vi "Get IP.vi"(8 "error in (no error)":errorcluster, 10 "ID":string, 11 "Guardian List in":refnum<class "Guardian List.lvclass">) -> (0 "error out":errorcluster, 2 "IP":string, 3 "Guardian List out":refnum<class "Guardian List.lvclass">)   [LabVIEW 2026, in "TALOS.lvlib" / "Classes.lvlib" / "Guardian List.lvclass"]
uses:
  Guardian List.lvclass
  Guardian List.lvclass/Guardian List.ctl
  Ancestor/Ancestor/Ancestor.lvclass/Ancestor.ctl
  FGV/Error Memory/Get Error Description.vi
  Support VIs/Get PC name.vi
  Ancestor/Ancestor/Read ID.vi
  Support VIs/Get Class Name.vi
  <vilib>/Utility/error.llb/Clear Errors.vi
  FGV/Error Memory/Error Memory Core.vi
  <vilib>/AdvancedString/Delimited String to 1D String Array.vi
  <vilib>/AdvancedString/Delimited String to 1D String Array (string).vi
  Support VIs/Circus Root Path.vi
  FGV/Error Memory/Error Crt Lvl checker.vi
  FGV/Error Memory/Error Memory Core.vi/40c8088d-b597-4017-91af-faa98e00292e.vi
  FGV/Error Memory/Error Memory Core.vi/d4a3ab98-063c-4e44-b43d-fbdcfe6c2be2.vi
  Support VIs/Global Memory.vi
  <vilib>/Utility/LVClass/Get LV Class Name.vi
  Support VIs/Is in Packed Library.vi
  Support VIs/TALOS Root path.vi
  Support VIs/Read CSV worksheet.vi
  Support VIs/Global Constants.vi
  <vilib>/Utility/error.llb/General Error Handler.vi
  Ancestor/Ancestor/Ancestor.lvclass
  <vilib>/Comparison/Equal/Equal Functor/Equal Functor.lvclass
  TALOS.lvlib
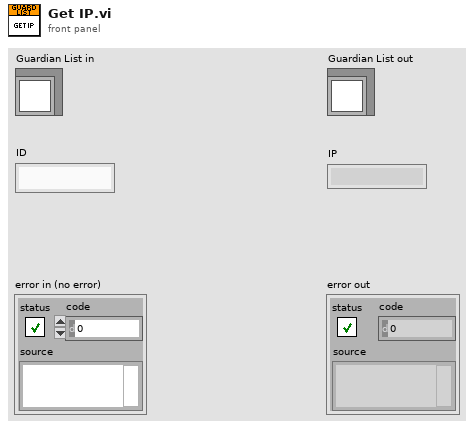
[diagram p1: front panel]
types:
  T1 = typedef "TALOS.lvlib/Classes.lvlib/Guardian List.lvclass/Guardian Properties.ctl" = cluster{"Alive":bool, "Last Seen":timestamp, "IP":string, "TCP Writer associated ID":string, "uS List received":bool, "Abort":bool, "Bearer":bool, "TCP Listener associated ID":string}
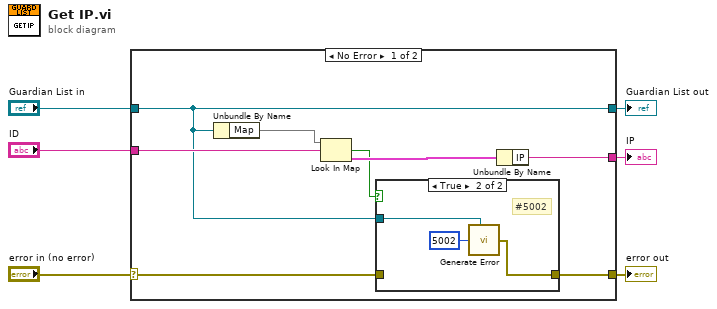
[diagram p0: block diagram]
diagram:
  n1 = case shown="No Error" "error in (no error)" {
    selector: "error in (no error)" -> [w9 w21]
    tunnel: [w8 w21] -> w5
    tunnel: [w7 w20] -> w3
    tunnel: "Guardian List in" -> [w7 w20]
    tunnel: "ID" -> [w13 w19]
    tunnel: [w11 w19] -> w1
    frame No Error {
      n2 = Unbundle By Name(w7) -> ("Map"=w14:map{string, T1})
      n3 = Look In Map(map=w14, key=w13) -> (key not found?=w10:bool, value=w12:T1)  [unwired: 1 in]
      n4 = case shown="True" w10 {
        tunnel: w9 -> [w15 _]
        tunnel: [w15 w16] -> w8
        tunnel: w7 -> [_ w17]
        frame False {
        }
        frame True {
          # "#5002"
          n5 = call "Generate Error.vi"("Class"=w17, "Error Code"=5002) -> ("error out"=w16:errorcluster)  [unwired: 5 in]
        }
      }
      n6 = Unbundle By Name(w12) -> ("IP"=w11:string)
    }
    frame Error {
    }
  }
  "error out" <- w5
  "Guardian List out" <- w3
  "IP" <- w1
